vi "ps control debug (fpga).vi"() -> ()   [LabVIEW 2019]
uses:
  <vilib>/eio/EIONode/EIONode.xnode
  <vilib>/rvi/eio/common/nirviEmuTemplateMethod_errors.vi
panel:
  out "PS Feedback 2":fxp<+/-,24,5>
  in  "PS Cmd 2":fxp<+/-,20,5>
  out "PS Feedback 1":fxp<+/-,24,5>
  in  "PS Cmd 1":fxp<+/-,20,5>
  in  "PWM Period (Ticks)":u32=400000
  in  "Duty (Ticks) 1":i32
  in  "Duty (Ticks) 2":i32
  in  "Duty (Ticks) 3":i32
  in  "Duty (Ticks) 4":i32
  in  "Duty (Ticks) 5":i32
  in  "Duty (Ticks) 6":i32
  in  "Loop Timer (uSec)":u32=1000
  out "Actual Loop Time":u32
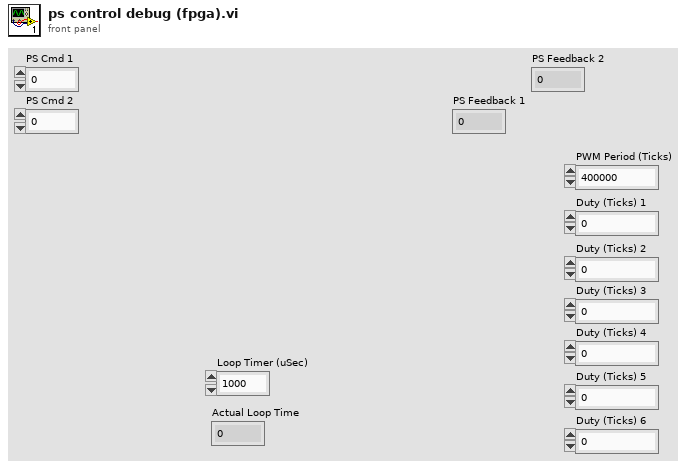
[diagram p1: front panel]
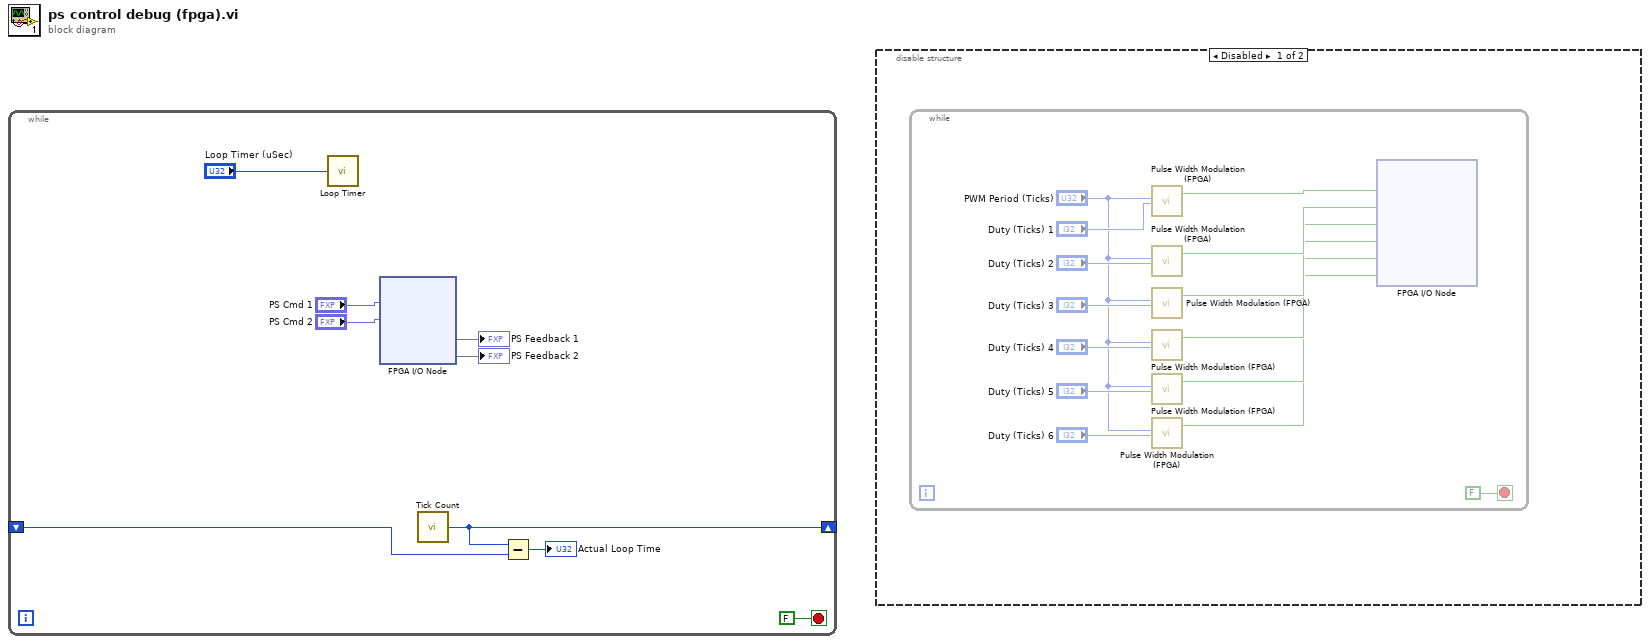
[diagram p0: block diagram]
diagram:
  n1 = while {
    shift-right: [w7] -> _
    shift-left: _ -> [w6]
    stop <- FALSE stop-if-true
    n2 = call "Loop Timer"("Count(uSec)"="Loop Timer (uSec)") -> ()  [unwired: 1 out]
    n3 = xnode "FPGA I/O Node"("AO0"="PS Cmd 1", "AO1"="PS Cmd 2") -> ("AI0"=→"PS Feedback 1", "AI1"=→"PS Feedback 2")  [unwired: 4 in, 4 out]
    n4 = call "Tick Count"() -> ("Tick Count(uSec)"=w7:u32)
    n5 = Subtract(x=w7, y=w6) -> (x-y=→"Actual Loop Time":u32)
  }
  n6 = disable-structure shown="Disabled" {
    frame Disabled {
      n7 = while {
        stop <- FALSE stop-if-true
        n8 = call "Pulse Width Modulation (FPGA).vi"("PWM Period (Ticks)"="PWM Period (Ticks)", "PWM Duty Cycle (Ticks)"="Duty (Ticks) 1") -> ("PWM DO"=w23:bool)  [unwired: 14 in, 3 out]
        n9 = call "Pulse Width Modulation (FPGA).vi"("PWM Period (Ticks)"="PWM Period (Ticks)", "PWM Duty Cycle (Ticks)"="Duty (Ticks) 2") -> ("PWM DO"=w20:bool)  [unwired: 14 in, 3 out]
        n10 = call "Pulse Width Modulation (FPGA).vi"("PWM Period (Ticks)"="PWM Period (Ticks)", "PWM Duty Cycle (Ticks)"="Duty (Ticks) 3") -> ("PWM DO"=w14:bool)  [unwired: 14 in, 3 out]
        n11 = call "Pulse Width Modulation (FPGA).vi"("PWM Period (Ticks)"="PWM Period (Ticks)", "PWM Duty Cycle (Ticks)"="Duty (Ticks) 4") -> ("PWM DO"=w13:bool)  [unwired: 14 in, 3 out]
        n12 = call "Pulse Width Modulation (FPGA).vi"("PWM Period (Ticks)"="PWM Period (Ticks)", "PWM Duty Cycle (Ticks)"="Duty (Ticks) 5") -> ("PWM DO"=w12:bool)  [unwired: 14 in, 3 out]
        n13 = call "Pulse Width Modulation (FPGA).vi"("PWM Period (Ticks)"="PWM Period (Ticks)", "PWM Duty Cycle (Ticks)"="Duty (Ticks) 6") -> ("PWM DO"=w11:bool)  [unwired: 14 in, 3 out]
        n14 = xnode "FPGA I/O Node"("RMC/DIO0"=w23, "RMC/DIO1"=w20, "RMC/DIO2"=w14, "RMC/DIO3"=w13, "RMC/DIO4"=w12, "RMC/DIO5"=w11) -> ()  [unwired: 7 in, 7 out]
      }
    }
    frame Enabled {
    }
  }
